vi "ImageEditModule.vi"(10 "skala szaroœci 2":u32(slide) scale=0.0..100.0, 11 "New Image":T1) -> (3 "Image 4":T1(plugin-control))   [LabVIEW 2023]
uses:
  <vilib>/vision/Image Controls.llb/IMAQ Image.ctl
panel:
  out "New Image 2":T1
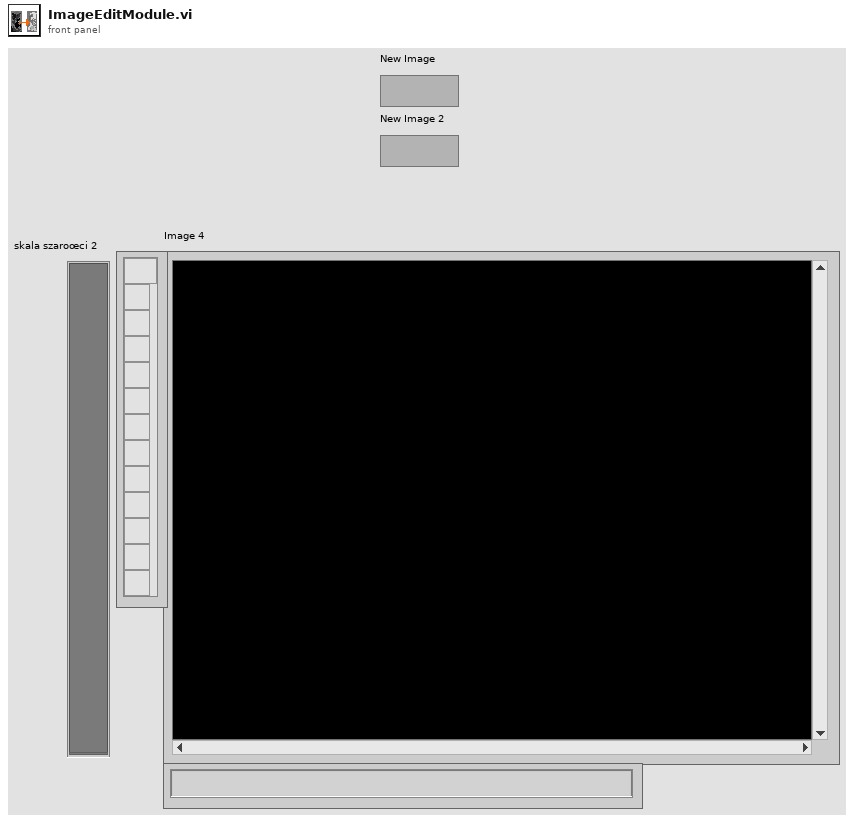
[diagram p1: front panel]
types:
  T1 = typedef "IMAQ Image.ctl" = refnum<image>
  T2 = typedef "Image Type" = u32
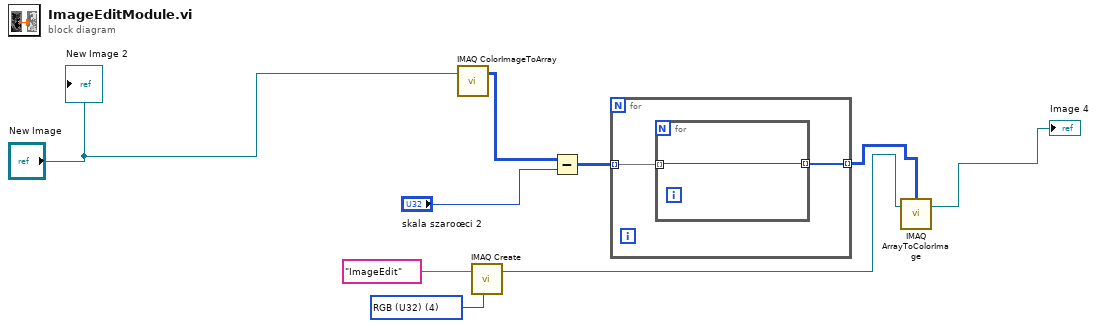
[diagram p0: block diagram]
diagram:
  w8 = T2 4 items=["Grayscale (U8)", "Grayscale (I16)", "Grayscale (SGL)", "Complex (CSG)", "RGB (U32)", "HSL (U32)", "RGB (U64)", "Grayscale (U16)"] ("Image Type")
  n1 = call "IMAQ ColorImageToArray"("Image"="New Image") -> ("Image Pixels (U32)"=w1:u32[][])  [unwired: 3 in, 2 out]
  n2 = call "IMAQ Create"("Image Name"="ImageEdit", "Image Type"=w8) -> ("New Image"=w4:T1)  [unwired: 3 in, 1 out]
  n3 = Subtract(x=w1, y="skala szaroœci 2") -> (x-y=w6:u32[][])
  n4 = for {
    tunnel: w6 -> [w11] mode=indexing
    tunnel: [w10] -> w5 mode=indexing
    n5 = for {
      tunnel: w11 -> [w12] mode=indexing
      tunnel: [w12] -> w10 mode=indexing
    }
  }
  n6 = call "IMAQ ArrayToColorImage"("Image Pixels (U32)"=w5, "Image"=w4) -> ("Image Out"=→"Image 4":T1)  [unwired: 3 in, 1 out]
  "New Image 2" <- "New Image"
